vi "UTILITY Delete Zeros.vi"(8 "Error In":errorcluster, 9 "Search # of Rows":i32, 10 "Data Array":dbl[](array[numeric]), 11 "Time Array":dbl[](array[numeric])) -> (0 "Error Out":errorcluster, 2 "Data Array Output":dbl[](array[numeric]), 3 "Time Array Output":dbl[](array[numeric]))   [LabVIEW 2016]
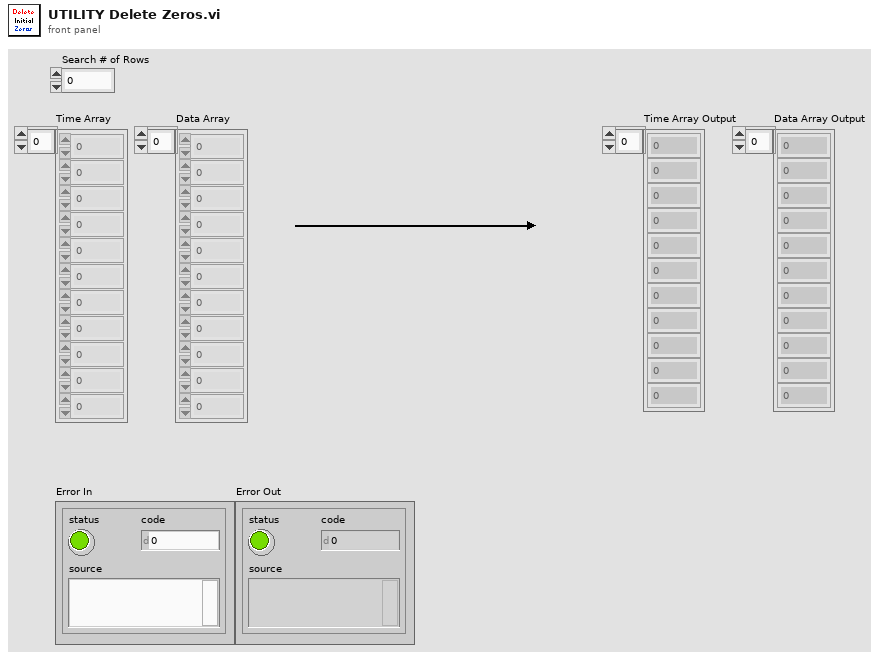
[diagram p1: front panel]
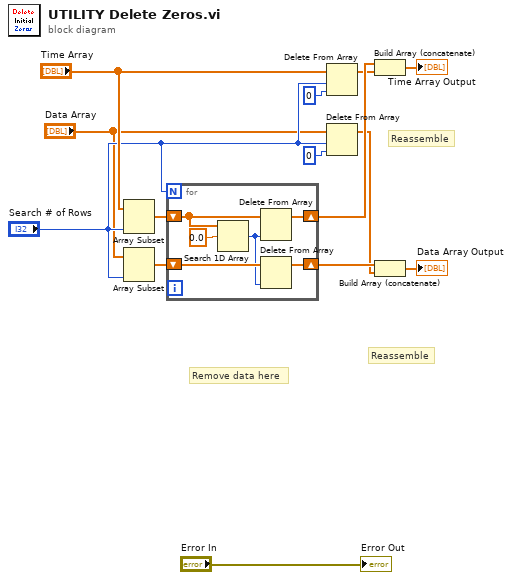
[diagram p0: block diagram]
diagram:
  # "Reassemble"
  # "Reassemble"
  # "Remove data here"
  n1 = Array Subset(array="Time Array", length="Search # of Rows") -> (w14:dbl[])  [unwired: 1 in]
  n2 = Array Subset(array="Data Array", length="Search # of Rows") -> (w13:dbl[])  [unwired: 1 in]
  n3 = for {
    N: "Search # of Rows" -> [_]
    shift-right: [w19] -> w12
    shift-left: w14 -> [w15]
    shift-right: [w17] -> w10
    shift-left: w13 -> [w18]
    n4 = Search 1D Array(1D array=w15, element=0.0) -> (index of element=w16:i32)  [unwired: 1 in]
    n5 = Delete From Array(array=w15, index=w16) -> (array with subset deleted=w19:dbl[])  [unwired: 1 in, 1 out]
    n6 = Delete From Array(array=w18, index=w16) -> (array with subset deleted=w17:dbl[])  [unwired: 1 in, 1 out]
  }
  n7 = Delete From Array(array="Time Array", length="Search # of Rows", index=0) -> (array with subset deleted=w4:dbl[])  [unwired: 1 out]
  n8 = Delete From Array(array="Data Array", length="Search # of Rows", index=0) -> (array with subset deleted=w5:dbl[])  [unwired: 1 out]
  n9 = Build Array (concatenate)(w12, w4) -> (→"Time Array Output":dbl[])
  n10 = Build Array (concatenate)(w10, w5) -> (→"Data Array Output":dbl[])
  "Error Out" <- "Error In"
